vi "Cannon Set.vi"(0 "Cannon Information":T1) -> ()   [LabVIEW 2012]
uses:
  <vilib>/Rock Robotics/WPI/Solenoid/WPI_SolenoidValue.ctl
  Cannon Global Data.vi
  <vilib>/Rock Robotics/WPI/Solenoid/WPI_SolenoidSetEnum.vi
  <vilib>/Rock Robotics/WPI/Compressor/WPI_CompressorGetSetRefNum.vi
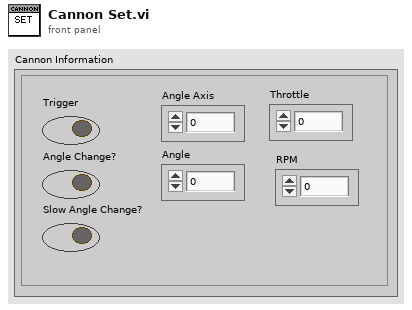
[diagram p1: front panel]
types:
  T1 = cluster{"RPM":dbl, "Trigger":bool, "Angle Axis":dbl, "Angle":dbl, "Throttle":dbl, "Slow Angle Change?":bool, "Angle Change?":bool}
  T2 = typedef "WPI_SolenoidValue.ctl" = enum16{"Off", "On", "Forward", "Reverse"}
  T3 = typedef "WPI_CompressorDevRef.ctl" = cluster{"DevStatus":errorcluster, "DigitalInputDevRef":T4, "RelayDevRef":T7}
  T4 = typedef "WPI_DigitalInputDevRef.ctl" = cluster{"DevStatus":errorcluster, "DIO Channel":T5, "Digital Module":T6}
  T5 = typedef "FPGA_DIOChannel.ctl" = enum8{"DIO 1", "DIO 2", "DIO 3", "DIO 4", "DIO 5", "DIO 6", "DIO 7", "DIO 8", "DIO 9", "DIO 10", "DIO 11", "DIO 12", "DIO 13", "DIO 14", "Invalid"}
  T6 = typedef "FPGA_TypedefDigitalModule.ctl" = enum16{"Digital Module 1", "Digital Module 2"}
  T7 = typedef "WPI_RelayDevRef.ctl" = cluster{"DevStatus":errorcluster, "Relay Channel":T8, "Digital Module":T6, "Relay Direction":T9}
  T8 = typedef "FPGA_DIORelayChannel.ctl" = enum8{"Relay 1", "Relay 2", "Relay 3", "Relay 4", "Relay 5", "Relay 6", "Relay 7", "Relay 8", "Invalid"}
  T9 = typedef "WPI_RelayDirection.ctl" = enum16{"Both directions", "Forward only", "Reverse only"}
  T10 = typedef "WPI_SolenoidDevRef.ctl" = cluster{"DevStatus":errorcluster, "Solenoid Module":T11, "Forward Solenoid Channel":T12, "Reverse Solenoid Channel":T12}
  T11 = typedef "FPGA_TypedefSolenoidModule.ctl" = enum16{"Solenoid Module 1", "Solenoid Module 2"}
  T12 = typedef "WPI_SolenoidChannel.ctl" = enum8{"Solenoid 1", "Solenoid 2", "Solenoid 3", "Solenoid 4", "Solenoid 5", "Solenoid 6", "Solenoid 7", "Solenoid 8", "Invalid"}
  T13 = typedef "WPI_RelayValue.ctl" = enum16{"Off", "On", "Forward", "Reverse"}
  T14 = typedef "WPI_MotorControlDeviceRef.ctl" = cluster{"DeviceStatus":errorcluster, "Type":enum16{"PWM", "CAN"}, "PWM":cluster{"Digital Module":T6, "PWM Channel":T15, "DeadBand":T16}, "CAN":cluster{"Device Number":u8, "Control Mode":T17, "Semaphore":T18, "Max Vout":dbl}, "Invert":bool, "TransformRef":T19, "InvTransformRef":T19}
  T15 = typedef "FPGA_DIOPWMChannel.ctl" = enum8{"PWM 1", "PWM 2", "PWM 3", "PWM 4", "PWM 5", "PWM 6", "PWM 7", "PWM 8", "PWM 9", "PWM 10", "Invalid"}
  T16 = typedef "WPI_PWMDeadband.ctl" = cluster{"Name":string, "maxPositivePwm":i32, "minPositivePwm":i32, "centerPwm":i32, "maxNegativePwm":i32, "minNegativePwm":i32, "angularRange":u16}
  T17 = typedef "WPI_CANJaguar_ControlMode.ctl" = enum8{"Percent VBus", "Current", "Speed", "Position", "Voltage"}
  T18 = typedef "Semaphore RefNum" = refnum<k1>
  T19 = typedef "WPI_PWMTransform_ConPane.ctl" = refnum<vi>
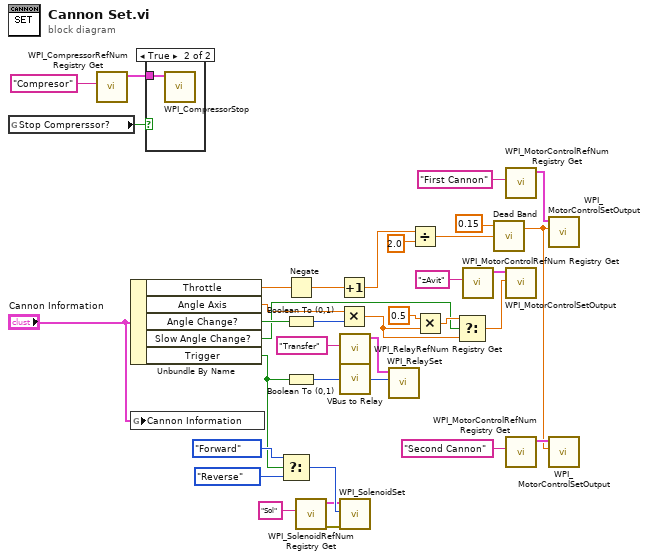
[diagram p0: block diagram]
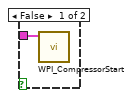
[diagram p2: hidden frame]
diagram:
  n1 = global read "Cannon Global Data.vi" "Stop Comprerssor?"() -> (w9:bool)
  n2 = call <vilib>:"WPI_CompressorRefNum Registry Get.vi"("refnum name"="Compresor") -> ("CompressorDevRef"=w7:T3)  [unwired: 9 in, 1 out]
  n3 = Unbundle By Name("Cannon Information") -> ("Throttle"=w27:dbl, "Angle Axis"=w4:dbl, "Angle Change?"=w22:bool, "Slow Angle Change?"=w21:bool, "Trigger"=w5:bool)
  n4 = global write "Cannon Global Data.vi" "Cannon Information"("Cannon Information") -> ()
  n5 = case shown="True" w9 {
    tunnel: w7 -> [w37 w38]
    frame False {
      n6 = call <vilib>:"WPI_CompressorStart.vi"("CompressorDevRef"=w37) -> ()  [unwired: 9 in, 2 out]
    }
    frame True {
      n7 = call <vilib>:"WPI_CompressorStop.vi"("CompressorDevRef"=w38) -> ()  [unwired: 9 in, 2 out]
    }
  }
  n8 = Select(t=WPI_SolenoidValue."Forward" ("Value"), s=w5, f=WPI_SolenoidValue."Reverse" ("Value")) -> (s? t:f=w12:T2)
  n9 = Negate(x=w27) -> (-x=w30:dbl)
  n10 = Boolean To (0,1)(Boolean=w22) -> (0, 1=w26:i16)
  n11 = Boolean To (0,1)(Boolean=w5) -> (0, 1=w2:i16)
  n12 = call <vilib>:"WPI_SolenoidRefNum Registry Get.vi"("refnum name"="Sol") -> ("error out"=w14:errorcluster, "SolenoidDevRef"=w11:T10)  [unwired: 9 in]
  n13 = Increment(x=w30) -> (x+1=w32:dbl)
  n14 = Multiply(x=w4, y=w26) -> (x*y=w24:dbl)
  n15 = call <vilib>:"WPI_RelayRefNum Registry Get.vi"("refnum name"="Transfer") -> ("RelayDevRef"=w16:T7)  [unwired: 9 in, 1 out]
  n16 = call "VBus to Relay.vi"("Motor VBus"=w2) -> ("RelayValue"=w3:T13)  [unwired: 3 in]
  n17 = call-poly <vilib>:"WPI_SolenoidSet.vi"("error in (no error)"=w14, "Value"=w12, "SolenoidDevRef"=w11) -> ()  [unwired: 9 out]
  n18 = call <vilib>:"WPI_RelaySet.vi"("RelayValue"=w3, "RelayDevRef"=w16) -> ()  [unwired: 8 in, 2 out]
  n19 = Divide(x=w32, y=2.0) -> (x/y=w28:dbl)
  n20 = Multiply(x=0.5, y=w24) -> (x*y=w25:dbl)
  n21 = Select(t=w25, s=w21, f=w24) -> (s? t:f=w6:dbl)
  n22 = call <vilib>:"WPI_MotorControlRefNum Registry Get.vi"("refnum name"="zAvit") -> ("MotorControlDevRef"=w19:T14)  [unwired: 9 in, 1 out]
  n23 = call "Dead Band.vi"("Axis 1 In"=w28, "Dead Band"=0.15) -> ("Axis 1 Out"=w18:dbl)  [unwired: 1 in, 1 out]
  n24 = call <vilib>:"WPI_MotorControlRefNum Registry Get.vi"("refnum name"="First Cannon") -> ("MotorControlDevRef"=w33:T14)  [unwired: 9 in, 1 out]
  n25 = call <vilib>:"WPI_MotorControlSetOutput.vi"("Output"=w6, "MotorControlDevRef"=w19) -> ()  [unwired: 7 in, 3 out]
  n26 = call <vilib>:"WPI_MotorControlRefNum Registry Get.vi"("refnum name"="Second Cannon") -> ("MotorControlDevRef"=w34:T14)  [unwired: 9 in, 1 out]
  n27 = call <vilib>:"WPI_MotorControlSetOutput.vi"("Output"=w18, "MotorControlDevRef"=w33) -> ()  [unwired: 7 in, 3 out]
  n28 = call <vilib>:"WPI_MotorControlSetOutput.vi"("Output"=w18, "MotorControlDevRef"=w34) -> ()  [unwired: 7 in, 3 out]
